vi "_TEST Sequences.vi"(4 "error in (no error)":errorcluster) -> (0 "error out":errorcluster)   [LabVIEW 2011]
uses:
  Sequence Record.ctl
  Sequence Fields.ctl
panel:
  out "Sequence Records":T1[](array[typedef])
  in  "Sort by":T2
  out "Sequence Record":T1
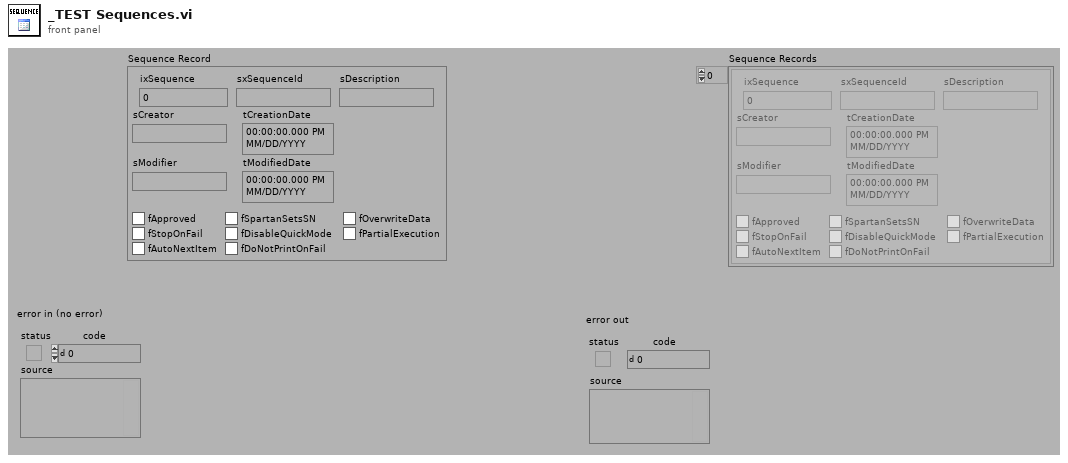
[diagram p1: front panel]
types:
  T1 = typedef "Sequence Record.ctl" = cluster{"ixSequence":i32, "sxSequenceId":string, "sDescription":string, "sCreator":string, "tCreationDate":timestamp, "sModifier":string, "tModifiedDate":timestamp, "fApproved":bool, "fSpartanSetsSN":bool, "fOverwriteData":bool, "fStopOnFail":bool, "fDisableQuickMode":bool, "fPartialExecution":bool, "fAutoNextItem":bool, "fDoNotPrintOnFail":bool}
  T2 = typedef "Sequence Fields.ctl" = enum32{"ixSequence", "sxSequenceId", "sDescription", "sCreator", "tCreationDate", "sModifier", "tModifiedDate", "fApproved", "fSpartanSetsSN", "fOverwriteData", "fStopOnFail", "fDisableQuickMode", "fPartialExecution", "fAutoNextItem"}
  T3 = typedef "Connection Refnum.ctl" = cluster{"Environment Handle":i32, "Connection Handle":i32}
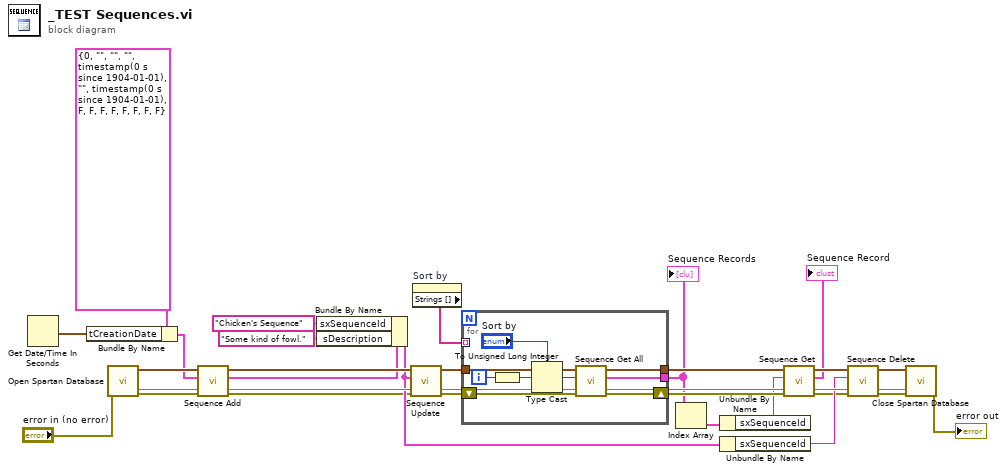
[diagram p0: block diagram]
diagram:
  n1 = Get Date/Time In Seconds() -> (seconds since 1Jan1904=w8:timestamp)
  n2 = Bundle By Name(cluster=T1 {"ixSequence"=0, "sxSequenceId"="", "sDescription"="", "sCreator"="", "tCreationDate"=timestamp(0 s since 1904-01-01), "sModifier"="", "tModifiedDate"=timestamp(0 s since 1904-01-01), "fApproved"=FALSE, "fSpartanSetsSN"=FALSE, "fOverwriteData"=FALSE, "fStopOnFail"=FALSE, "fDisableQuickMode"=FALSE, "fPartialExecution"=FALSE, "fAutoNextItem"=FALSE, "fDoNotPrintOnFail"=FALSE} ("Sequence Record"), "tCreationDate"=w8) -> (w6:T1)
  n3 = call "Open Spartan Database.vi"("error in (no error)"="error in (no error)") -> ("error out"=w25:errorcluster, "Connection Refnum"=w24:T3, 4:w26)  [unwired: 1 in, 7 out]
  n4 = call "Sequence Add.vi"("error in (no error)"=w25, "Sequence Record"=w6, "Connection Refnum"=w24) -> ("error out"=w20:errorcluster, "New Sequence Record"=w5:T1, "Connection Refnum"=w22:T3)  [unwired: 6 out]
  n5 = Bundle By Name(cluster=w5, "sxSequenceId"="Chicken's Sequence" ("Name"), "sDescription"="Some kind of fowl." ("Name")) -> (w21:T1)
  n6 = call "Sequence Update.vi"("error in (no error)"=w20, "Sequence Record"=w21, "Connection Refnum"=w22) -> ("error out"=w17:errorcluster, "Connection Refnum"=w16:T3)  [unwired: 7 out]
  n7 = property on="Sort by" class="Enum (strict)"() -> ("Strings []"=w9:string[])  [unwired: 2 in, 2 out]
  n8 = for {
    shift-right: [w36] -> w14
    shift-left: w17 -> [w33]
    tunnel: w16 -> [w37]
    tunnel: [w35] -> w13
    tunnel: [w34] -> w15
    tunnel: w9 -> [_] mode=indexing
    i -> [w30]
    n9 = To Unsigned Long Integer(number=w30) -> (unsigned 32bit integer=w29:u32)
    n10 = Type Cast(type="Sort by", x=w29) -> (*(type *) &x=w31:T2)
    n11 = call "Sequence Get All.vi"("error in (no error)"=w33, "Sort by (sxSequenceId)"=w31, "Connection Refnum"=w37) -> ("error out"=w36:errorcluster, "Sequence Records"=w35:T1[], "Connection Refnum"=w34:T3)  [unwired: 1 in, 5 out]
  }
  "Sequence Records" <- w13
  n12 = Index Array(array=w13) -> (element=w12:T1)  [unwired: 1 in]
  n13 = Unbundle By Name(w12) -> ("sxSequenceId"=w11:string)
  n14 = Unbundle By Name(w21) -> ("sxSequenceId"=w23:string)
  n15 = call "Sequence Get.vi"("error in (no error)"=w14, "sxSequenceId (\"\")"=w11, "Connection Refnum"=w15) -> ("error out"=w18:errorcluster, "Sequence Record"=→"Sequence Record":T1, "Connection Refnum"=w19:T3)  [unwired: 6 out]
  n16 = call "Sequence Delete.vi"("error in (no error)"=w18, "Sequence ID"=w23, "Connection Refnum"=w19) -> ("error out"=w28:errorcluster, "Connection Refnum"=w27:T3)  [unwired: 7 out]
  n17 = call "Close Spartan Database.vi"("Force Close? (f)"=w26, "error in (no error)"=w28, "Connection Refnum"=w27) -> ("error out"=→"error out":errorcluster)  [unwired: 1 in, 7 out]
